vi "CreatFromSerialNumNoRaw.vi"(8 "error in (no error)":errorcluster, 11 "APD Serial #":string) -> (0 "error out":errorcluster, 3 "APDClass out":refnum<class "APDClass.lvclass">)   [LabVIEW 2020, in "APDClass.lvclass"]
uses:
  APDClass.lvclass
  iRFData.ctl
  GainData.ctl
panel:
  out "GainRawTempError":errorcluster
  out "GainData":T1
  out "Mesurment date":string
  out "iRF Data":T2
  out "Waveform Graph":dbl[][](graph)
  out "Gain Curve":cluster{dbl[], dbl[]}(graph)
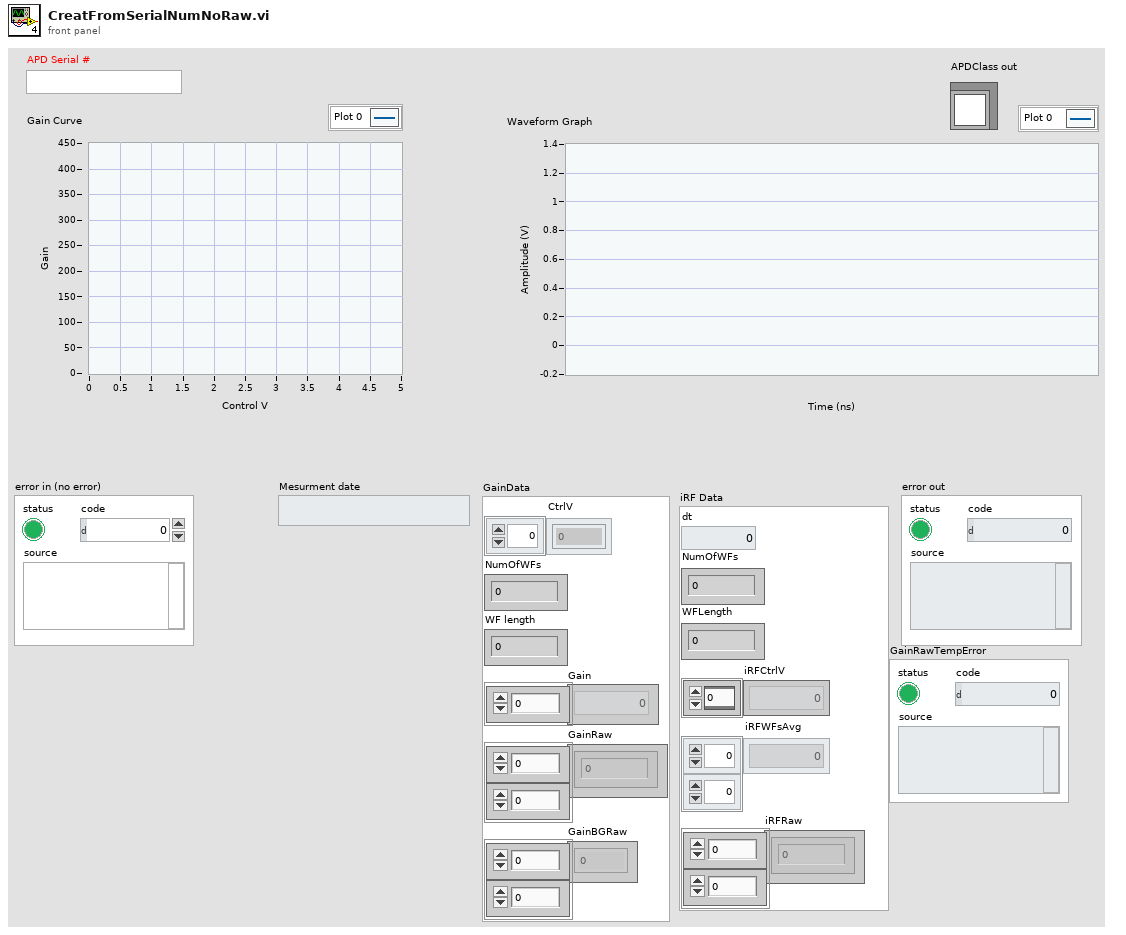
[diagram p1: front panel]
types:
  T1 = typedef "GainData.ctl" = cluster{"CtrlV":dbl[], "NumOfWFs":i32, "WF length":i32, "Gain":dbl[], "GainRaw":dbl[][], "GainBGRaw":dbl[][]}
  T2 = typedef "iRFData.ctl" = cluster{"dt":dbl, "NumOfWFs":i32, "WFLength":i32, "iRFCtrlV":dbl[], "iRFWFsAvg":dbl[][], "iRFRaw":dbl[][]}
  T3 = enum16{"open", "open or create", "create or replace", "create", "open (read-only)"}
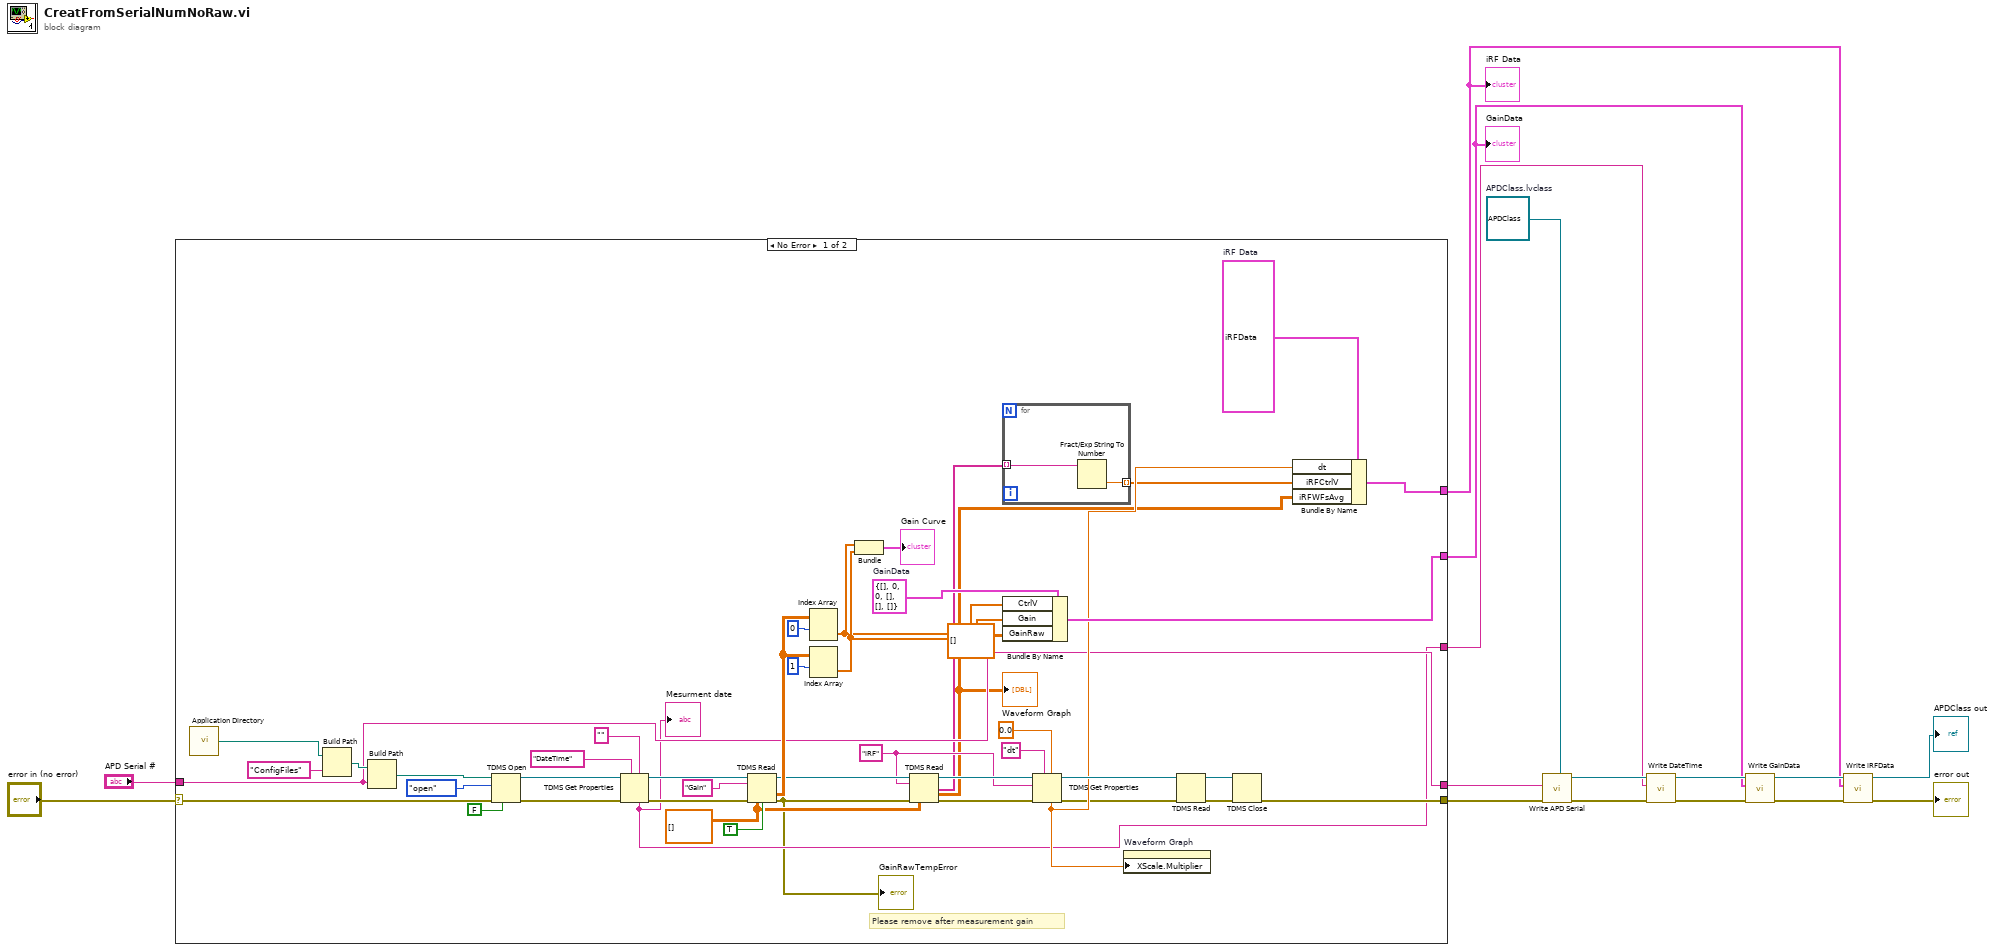
[diagram p0: block diagram]
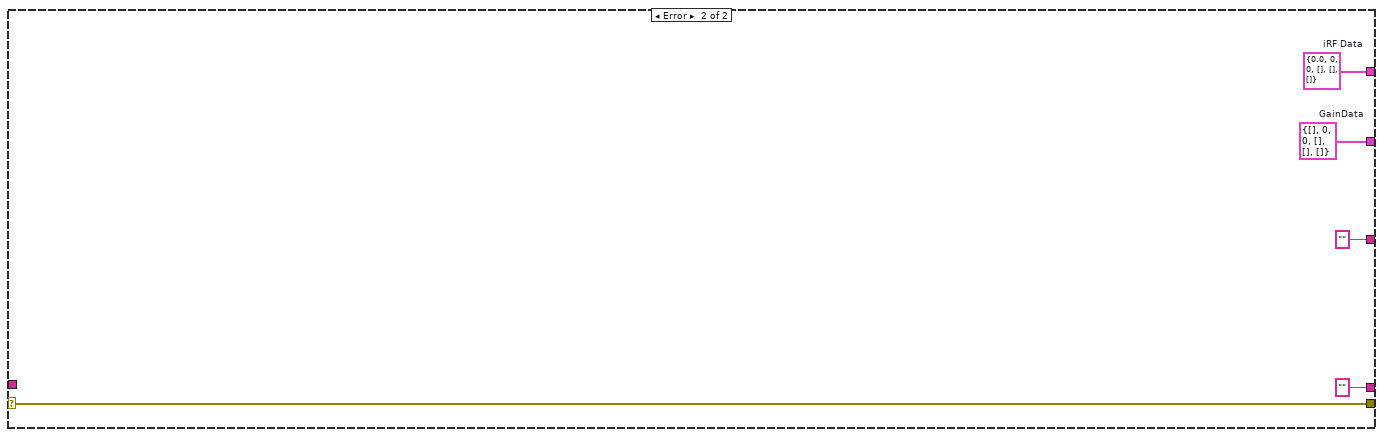
[diagram p2: hidden frame]
diagram:
  w14 = refnum<class "APDClass.lvclass"> refnum  # APDClass.lvclass
  n1 = case shown="No Error" "error in (no error)" {
    selector: "error in (no error)" -> [w40 w68]
    tunnel: [w39 w68] -> w12
    tunnel: "APD Serial #" -> [w35 _]
    tunnel: [w38 w67] -> w10
    tunnel: [w37 w64] -> w1
    tunnel: [w35 "" ("APD Serial #")] -> w13
    tunnel: [w28 ""] -> w2
    frame No Error {
      w27 = T1 {"CtrlV"=[], "NumOfWFs"=0, "WF length"=0, "Gain"=[], "GainRaw"=[], "GainBGRaw"=[]}  # GainData
      w45 = T2 {"dt"=0.0, "NumOfWFs"=0, "WFLength"=0, "iRFCtrlV"=[0.0, 0.1, 0.2, 0.30000000000000004, 0.4, 0.5, 0.6000000000000001, 0.7000000000000001, 0.8, 0.9, 1.0, 1.1, 1.2000000000000002, 1.3, 1.4000000000000001, 1.5, 1.6, 1.7000000000000002, 1.8, 1.9000000000000001, 2.0, 2.1, 2.2, 2.3000000000000003, 2.4000000000000004, 2.5, 2.6, 2.7, 2.8000000000000003, 2.9000000000000004, 3.0, 3.1, 3.2, 3.3000000000000003, 3.4000000000000004, 3.5, 3.6, 3.7, 3.8000000000000003, 3.9000000000000004, 4.0, 4.1000000000000005, 4.2, 4.3, 4.4, 4.5, 4.6000000000000005], "iRFWFsAvg"=array47x600[28200 elements], "iRFRaw"=[]}  # iRF Data
      w43 = "iRF" ("group name in (Untitled)")
      w19 = dbl[][] []
      # "Please remove after measurement gain"
      n2 = call <vilib>:"Application Directory.vi"() -> ("Application Directory"=w61:path)
      n3 = Build Path(base path=w61, name or relative path="ConfigFiles") -> (appended path=w59:path)
      n4 = Build Path(base path=w59, name or relative path=w35) -> (appended path=w58:path)
      n5 = TDMS Open(6:FALSE ("disable buffering? (T)"), 8:w40, 10:T3."open" ("operation (0:open)"), 11:w58) -> (0:w33:errorcluster, 3:w34:refnum<k34>)  [unwired: 3 in]
      n6 = TDMS Get Properties(5:"", 7:"DateTime" ("property name"), 8:w33, 11:w34) -> (0:w29:errorcluster, 3:w30:refnum<k34>, 4:w28:string)  [unwired: 2 in, 3 out]
      "Mesurment date" <- w28
      n7 = TDMS Read(0:w30, 5:"Gain" ("group name in"), 11:w29, 12:w19, 13:TRUE ("return channels in file order? (F)")) -> (4:w49:refnum<k34>, 10:w52:dbl[][], 15:w18:errorcluster)  [unwired: 3 in, 3 out]
      "GainRawTempError" <- w18
      n8 = Index Array(array=w52, index (row)=0) -> (element=w23:dbl[])  [unwired: 1 in]
      n9 = Index Array(array=w52, index (row)=1) -> (element=w46:dbl[])  [unwired: 1 in]
      n10 = Bundle(w23, w46) -> (→"Gain Curve":cluster{dbl[], dbl[]})  [unwired: 1 in]
      n11 = TDMS Read(0:w49, 5:w43, 11:w18, 12:w19) -> (4:w48:refnum<k34>, 8:w26:string[], 10:w25:dbl[][], 15:w47:errorcluster)  [unwired: 4 in, 2 out]
      "Waveform Graph" <- w25
      n12 = for {
        tunnel: w26 -> [w63] mode=indexing
        tunnel: [w62] -> w24 mode=indexing
        n13 = Fract/Exp String To Number(string=w63) -> (number=w62:dbl)  [unwired: 3 in, 1 out]
      }
      n14 = Bundle By Name(cluster=w27, "CtrlV"=w23, "Gain"=w46, "GainRaw"=dbl[][] []) -> (w37:T1)
      n15 = TDMS Get Properties(5:0.0, 7:"dt", 8:w47, 10:w43, 11:w48) -> (0:w21:errorcluster, 3:w44:refnum<k34>, 4:w36:dbl)  [unwired: 1 in, 3 out]
      n16 = property on="Waveform Graph" class="WFGraph (strict)"("XScale.Multiplier"=w36) -> ()  [unwired: 2 in, 2 out]
      n17 = TDMS Read(0:w44, 11:w21) -> (4:w22:refnum<k34>, 15:w20:errorcluster)  [unwired: 6 in, 4 out]
      n18 = TDMS Close(8:w20, 11:w22) -> (0:w39:errorcluster)  [unwired: 1 out]
      n19 = Bundle By Name(cluster=w45, "dt"=w36, "iRFCtrlV"=w24, "iRFWFsAvg"=w25) -> (w38:T2)
    }
    frame Error {
      w64 = T1 {"CtrlV"=[], "NumOfWFs"=0, "WF length"=0, "Gain"=[], "GainRaw"=[], "GainBGRaw"=[]}  # GainData
      w67 = T2 {"dt"=0.0, "NumOfWFs"=0, "WFLength"=0, "iRFCtrlV"=[], "iRFWFsAvg"=[], "iRFRaw"=[]}  # iRF Data
    }
  }
  "iRF Data" <- w10
  "GainData" <- w1
  n20 = call-dynamic "Write APD Serial.vi"("error in (no error)"=w12, "APD Serial #"=w13, "APDClass in"=w14) -> ("error out"=w5:errorcluster, "APDClass out"=w6:refnum<class "APDClass.lvclass">)  [unwired: 7 in]
  n21 = call-dynamic "Write DateTime.vi"("error in (no error)"=w5, "DateTime"=w2, "APDClass in"=w6) -> ("error out"=w3:errorcluster, "APDClass out"=w4:refnum<class "APDClass.lvclass">)  [unwired: 7 in]
  n22 = call-dynamic "Write GainData.vi"("error in (no error)"=w3, "GainData"=w1, "APDClass in"=w4) -> ("error out"=w9:errorcluster, "APDClass out"=w11:refnum<class "APDClass.lvclass">)  [unwired: 7 in]
  n23 = call-dynamic "Write iRFData.vi"("error in (no error)"=w9, "iRFData"=w10, "APDClass in"=w11) -> ("error out"=→"error out":errorcluster, "APDClass out"=→"APDClass out":refnum<class "APDClass.lvclass">)  [unwired: 7 in]
